vi "Stop Motion.vi"(8 "error in (no error)":errorcluster, 11 "2-Axis Stage in":refnum<class "XY Stage Controller.lvclass">) -> (0 "error out":errorcluster, 3 "2-Axis Stage out":refnum<class "XY Stage Controller.lvclass">)   [LabVIEW 2022 SP3, in "XY Stage Controller.lvclass"]
uses:
  XY Stage Controller.lvclass
  XY Stage Controller.lvclass/XY Stage Controller.ctl
  Process Framework/Process State Data/Process State Data.lvclass/Process State Data.ctl
  Process Framework/Interlock Q Class/Interlock Q Class.lvclass/Interlock Q Class.ctl
  <vilib>/ActorFramework/Message Enqueuer/Message Enqueuer.lvclass/Message Enqueuer.ctl
  Process Framework/Process State Data/Accessor/Write Abort.vi
  <vilib>/ActorFramework/Message Enqueuer/Enqueue.vi
  XY Stage Process/XY Stage Process/XY Stage Process Messages/Stop Motion Msg/Stop Motion Msg.lvclass
  C:/Program Files/National Instruments/LabVIEW 2022/vi.lib/ActorFramework/Message/Message.lvclass
  <vilib>/ActorFramework/Message Priority Queue/Priority Enqueue.vi
  <vilib>/ActorFramework/Message Enqueuer/Message Enqueuer.lvclass
  Process Framework/Process State Data/Process State Data.lvclass
  Process Framework/Interlock Q Class/Interlock Q Class.lvclass
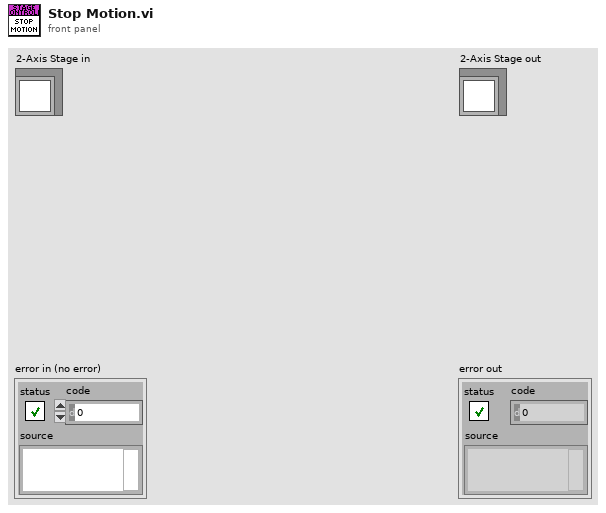
[diagram p1: front panel]
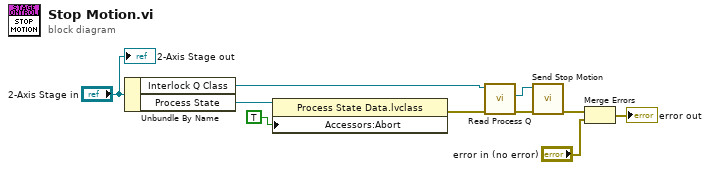
[diagram p0: block diagram]
diagram:
  n1 = Unbundle By Name("2-Axis Stage in") -> ("Interlock Q Class"=w7:refnum<class "Interlock Q Class.lvclass">, "Process State"=w9:refnum<data-value>)
  n2 = property class="Process State Data.lvclass"(reference=w9, "Accessors:Abort"=TRUE ("Abort")) -> (error out=w2:errorcluster)  [unwired: 1 in, 1 out]
  n3 = call "Read Process Q.vi"("error in (no error)"=w2, "Interlock Q Class in"=w7) -> ("error out"=w3:errorcluster, "Actor Framework:Message Enqueuer"=w6:refnum<class "Message Enqueuer.lvclass">)  [unwired: 7 in, 1 out]
  n4 = call "Send Stop Motion.vi"("error in (no error)"=w3, "Message Enqueuer"=w6) -> ("error out"=w4:errorcluster)  [unwired: 8 in, 1 out]
  n5 = Merge Errors(w4, "error in (no error)") -> (→"error out":errorcluster)
  "2-Axis Stage out" <- "2-Axis Stage in"
